vi "Test Insert Tables with data.vi"(11 "Test Case In":refnum<class "Test Open Xml.lvclass">) -> (0 "error out":errorcluster, 3 "Test Case Out":refnum<class "Test Open Xml.lvclass">)   [LabVIEW 2020, in "Test Open Xml.lvclass"]
uses:
  Test Open Xml.lvclass
  Source/Open Xml.lvlib
  0a0d70f3-36fe-46ba-8b3e-e6c07e708d9f.vi
panel:
  out "Sheet Name":string
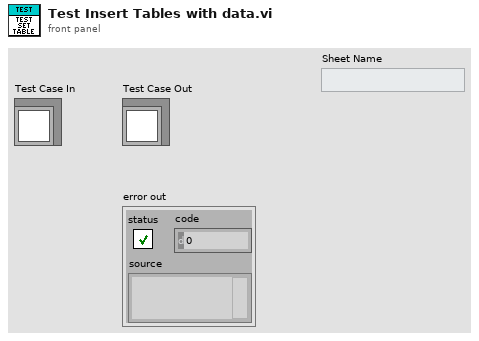
[diagram p1: front panel]
types:
  T1 = cluster{"Sheet Name":string, "Name":string, "Display Name":string, "Range or Cell Address":string}
  T2 = cluster{"Sheet Name":string, "Name":string, "Display Name":string, "Range":string}
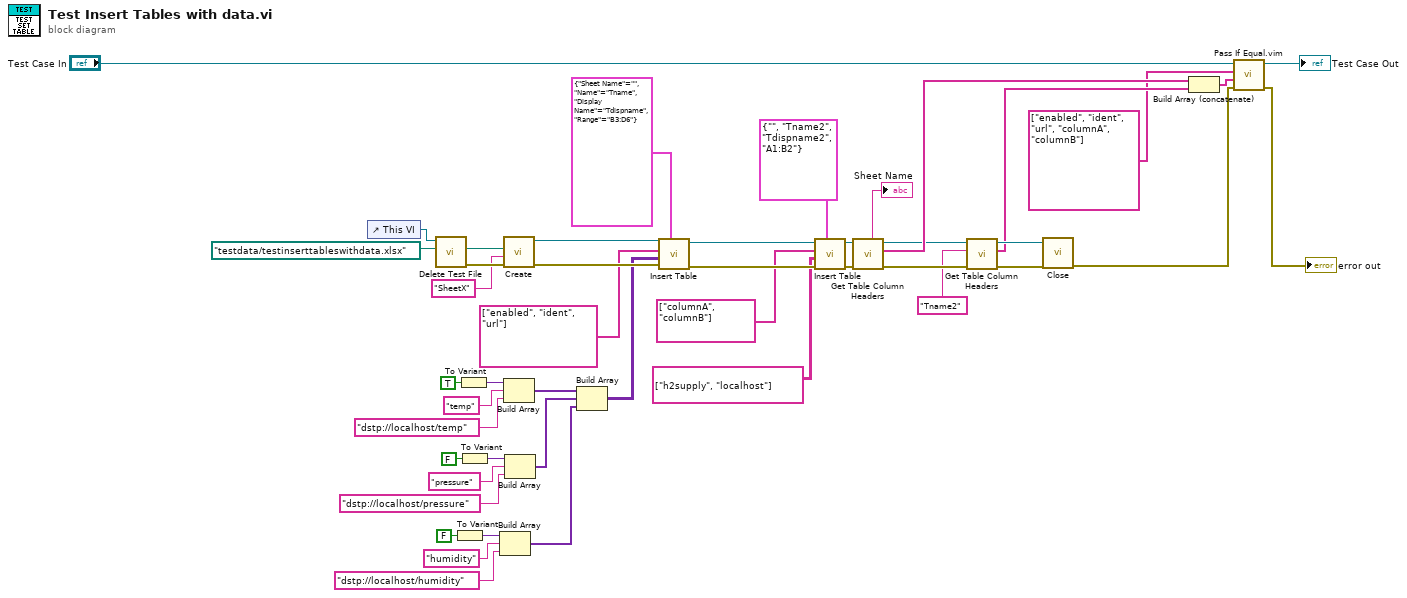
[diagram p0: block diagram]
diagram:
  n1 = control-ref of="This VI"() -> (w36:refnum<vi>)
  n2 = call "Delete Test File.vi"("name or relative path"=path "testdata/testinserttableswithdata.xlsx", "VI in"=w36) -> ("error out"=w37:errorcluster, "deleted path"=w38:path)  [unwired: 8 in]
  n3 = To Variant(anything=FALSE) -> (Variant=w7:variant)
  n4 = To Variant(anything=TRUE) -> (Variant=w16:variant)
  n5 = To Variant(anything=FALSE) -> (Variant=w10:variant)
  n6 = Build Array(w7, "humidity", "dstp://localhost/humidity") -> (w3:variant[])
  n7 = call "Create.vi"("error in"=w37, "SheetName"="SheetX", "Path"=w38) -> ("error out"=w33:errorcluster, "SpreadsheetDoc"=w34:refnum<k24>)  [unwired: 7 in]
  n8 = Build Array(w16, "temp", "dstp://localhost/temp") -> (w13:variant[])
  n9 = Build Array(w10, "pressure", "dstp://localhost/pressure") -> (w4:variant[])
  n10 = Build Array(w13, w4, w3) -> (w2:variant[][])
  n11 = call "Insert Table.vi"("Location"=T2 {"Sheet Name"="", "Name"="Tname", "Display Name"="Tdispname", "Range"="B3:D6"}, "error in"=w33, "Cell Values"=w2, "Header Names"=string[] ["enabled", "ident", "url"], "SpreadsheetDoc in"=w34) -> ("error out"=w40:errorcluster, "SpreadsheetDoc out"=w28:refnum<k24>)  [unwired: 5 in]
  n12 = call "Insert Table.vi"("Location"=T1 {"Sheet Name"="", "Name"="Tname2", "Display Name"="Tdispname2", "Range or Cell Address"="A1:B2"}, "error in"=w40, "Cell Values"=string[][] [["h2supply", "localhost"]], "Header Names"=string[] ["columnA", "columnB"], "SpreadsheetDoc in"=w28) -> ("error out"=w29:errorcluster, "SpreadsheetDoc out"=w27:refnum<k24>)  [unwired: 5 in]
  n13 = call "Get Table Column Headers.vi"("error in"=w29, "SpreadsheetDoc in"=w27) -> ("error out"=w42:errorcluster, "Headers"=w41:string[], "SpreadsheetDoc out"=w23:refnum<k24>, "Sheet Name out"=→"Sheet Name":string)  [unwired: 6 in]
  n14 = call "Get Table Column Headers.vi"("error in"=w42, "Table Name"="Tname2", "SpreadsheetDoc in"=w23) -> ("error out"=w24:errorcluster, "Headers"=w20:string[], "SpreadsheetDoc out"=w22:refnum<k24>)  [unwired: 5 in, 1 out]
  n15 = call "Close.vi"("error in"=w24, "SpreadsheetDoc"=w22) -> ("error out"=w43:errorcluster)  [unwired: 9 in]
  n16 = Build Array (concatenate)(w41, w20) -> (w21:string[])
  n17 = call "Pass If Equal.vim"("error in (no error)"=w43, "Actual"=w21, "Expected"=string[] ["enabled", "ident", "url", "columnA", "columnB"] ("Headers"), "LUnit Test Case In"="Test Case In") -> ("error out"=→"error out":errorcluster, "LUnit Test Case Out"=→"Test Case Out":refnum<class "Test Open Xml.lvclass">)  [unwired: 6 in]
